vi "Read ADC.vi"(8 "error in (no error)":errorcluster, 10 "ADC Channel":dbl, 11 "object in":refnum<class "Simulado.lvclass">) -> (0 "error out":errorcluster, 3 "object out":refnum<class "Simulado.lvclass">)   [LabVIEW 2020, in "Simulado.lvclass"]
uses:
  Simulado.lvclass
  Simulado.lvclass/Simulado.ctl
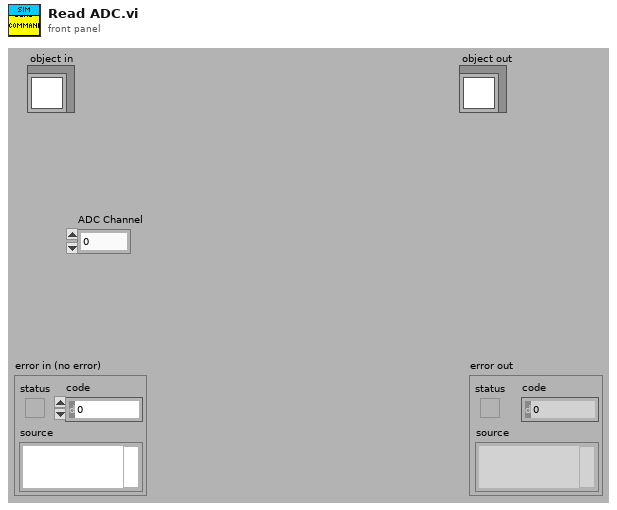
[diagram p1: front panel]
types:
  T1 = enum16{"Get Parameters", "Set Parameters", "Reset"}
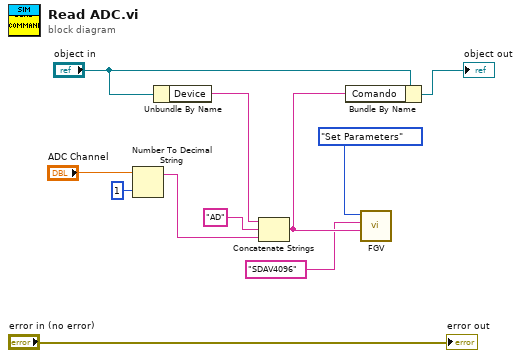
[diagram p0: block diagram]
diagram:
  n1 = Number To Decimal String(number="ADC Channel", width (-)=i16 1) -> (decimal integer string=w4:string)
  n2 = Unbundle By Name("object in") -> ("Device"=w8:string)
  n3 = Concatenate Strings(w8, "AD" ("string"), w4) -> (w7:string)
  n4 = Bundle By Name(cluster="object in", "Comando"=w7) -> (→"object out":refnum<class "Simulado.lvclass">)
  n5 = call "FGV.vi"("Comandos"=w7, "Respuestas"="SDAV4096", "Función"=T1."Set Parameters") -> ()  [unwired: 8 in, 1 out]
  "error out" <- "error in (no error)"
